vi "test Loopback with Scaled Parameters.vi"(8 "error in":errorcluster, 11 "TestCase in":refnum<class "Loopback.lvclass">) -> (0 "error out":errorcluster, 3 "TestCase out":refnum<class "Loopback.lvclass">)   [LabVIEW 2020, in "Loopback.lvclass"]
uses:
  Loopback.lvclass
  C:/dev/niveristand-custom-device-testing-tools/VeriStandTestCase/VeriStandTestCase.lvclass
  Loopback.lvclass/Loopback.ctl
  485b7c2b-8320-4722-9ec7-d01f27c65546.vi
  <vilib>/NI VeriStand/Execution/Workspace/NI VeriStand - Get Multiple Channel Values.vi
  <vilib>/NI VeriStand/Execution/Workspace/NI VeriStand - Set Multiple Channel Values.vi
  <vilib>/addons/_JKI Toolkits/VI Tester/TestCase.llb/TestCase.lvclass
  <vilib>/NI VeriStand/Execution/Workspace/NI_VS Workspace ExecutionAPI.lvlib
  C:/Program Files (x86)/National Instruments/LabVIEW 2020/vi.lib/addons/_JKI Toolkits/VI Tester/TestCase.llb/TestCase.lvclass
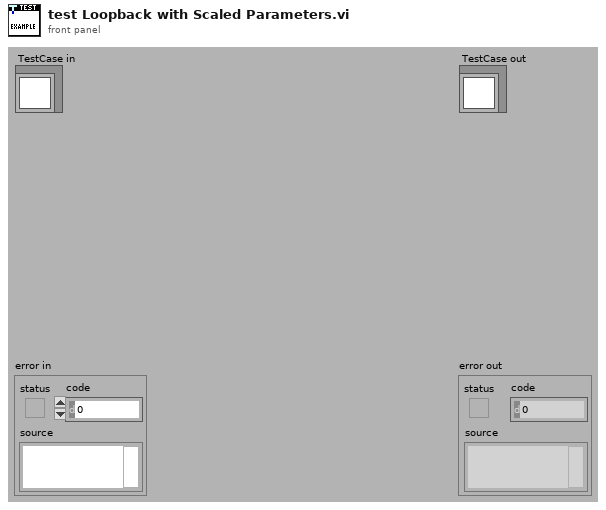
[diagram p1: front panel]
types:
  T1 = typedef "NI_VS Workspace ExecutionAPI.lvlib/WorkspaceAPI.ctl" = refnum<k24>
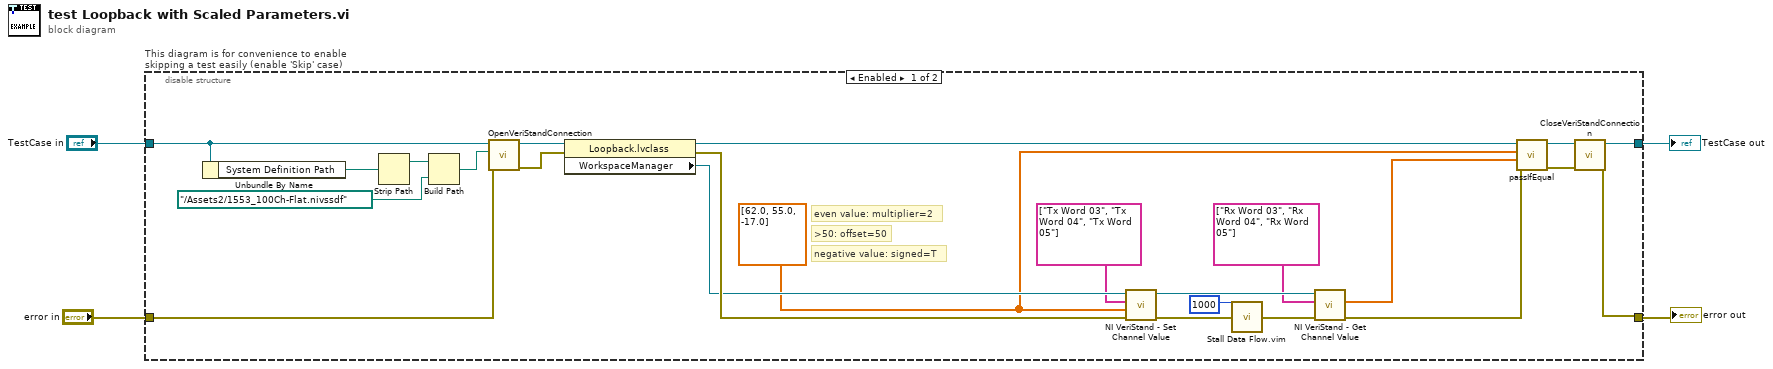
[diagram p0: block diagram]
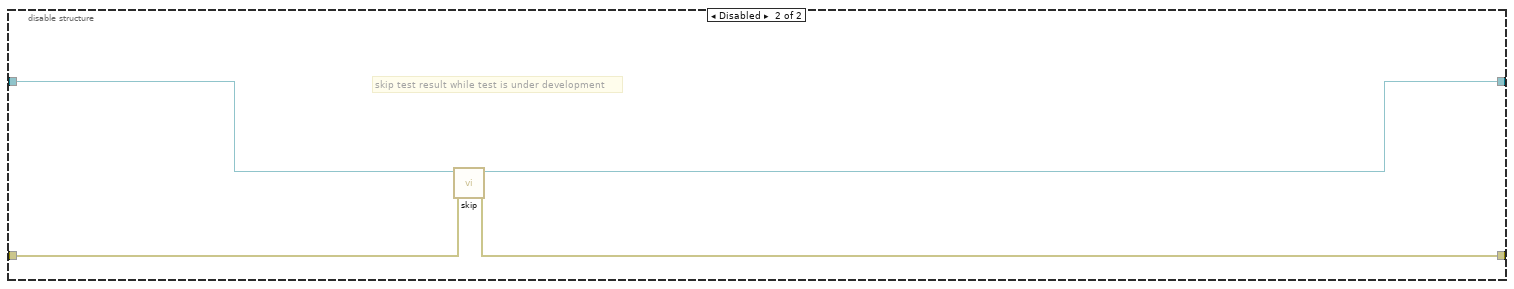
[diagram p2: hidden frame]
diagram:
  n1 = disable-structure "This diagram is for convenience to enable skipping a test easily (enable 'Skip' case)" shown="Enabled" {
    disable-tunnel: "TestCase in" -> [w23 w32]
    disable-tunnel: [w9 w30] -> w1
    disable-tunnel: [w5 w31] -> w3
    disable-tunnel: "error in" -> [w24 w29]
    frame Enabled {
      w6 = dbl[] [62.0, 55.0, -17.0] ("Values")
      # "negative value: signed=T"
      # ">50: offset=50"
      # "even value: multiplier=2"
      n2 = Unbundle By Name(w23) -> ("System Definition Path"=w27:path)
      n3 = Strip Path(path=w27) -> (stripped path=w26:path)  [unwired: 1 out]
      n4 = Build Path(base path=w26, name or relative path=path "../Assets2/1553_100Ch-Flat.nivssdf") -> (appended path=w25:path)
      n5 = call-dynamic "OpenVeriStandConnection.vi"("error in (no error)"=w24, "System Definition File"=w25, "VeriStand Test Case in"=w23) -> ("error out"=w20:errorcluster, "VeriStand Test Case out"=w22:refnum<class "Loopback.lvclass">)  [unwired: 6 in, 1 out]
      n6 = property class="Loopback.lvclass"(reference=w22, error in=w20) -> (reference out=w21:refnum<class "Loopback.lvclass">, error out=w15:errorcluster, "WorkspaceManager"=w13:T1)
      n7 = call-poly <vilib>:"NI VeriStand - Set Channel Value.vi"("error in (no error)"=w15, "Values"=w6, "Channels"=string[] ["Tx Word 03", "Tx Word 04", "Tx Word 05"], "WorkspaceManager in"=w13) -> ("error out"=w17:errorcluster, "WorkspaceManager out"=w19:T1)  [unwired: 6 in]
      n8 = call "Stall Data Flow.vim"("value in"=w17, "milliseconds to wait"=u32 1000) -> ("value out"=w18:errorcluster)  [unwired: 1 out]
      n9 = call-poly <vilib>:"NI VeriStand - Get Channel Value.vi"("error in (no error)"=w18, "Channels"=string[] ["Rx Word 03", "Rx Word 04", "Rx Word 05"], "WorkspaceManager in"=w19) -> ("error out"=w14:errorcluster, "Values"=w7:dbl[])  [unwired: 6 in, 1 out]
      n10 = call-dynamic "passIfEqual.vi"("error in (no error)"=w14, "y"=w7, "x"=w6, "TestCase in"=w21) -> ("error out"=w8:errorcluster, "TestCase out"=w10:refnum<class "Loopback.lvclass">)  [unwired: 6 in]
      n11 = call-dynamic "CloseVeriStandConnection.vi"("error in (no error)"=w8, "VeriStand Test Case in"=w10) -> ("error out"=w5:errorcluster, "VeriStand Test Case out"=w9:refnum<class "Loopback.lvclass">)  [unwired: 8 in]
    }
    frame Disabled {
      # "skip test result while test is under development"
      n12 = call <vilib>:"skip.vi"("error in (no error)"=w29, "TestCase in"=w32) -> ("error out"=w31:errorcluster, "TestCase out"=w30:refnum<class "Loopback.lvclass">)  [unwired: 8 in]
    }
  }
  "error out" <- w3
  "TestCase out" <- w1
